vi "VISA Group WR.vi"(8 "error in (no error)":errorcluster, 10 "Array in":string[](array[string]), 11 "VISA Refnum in":refnum<visa-resource-name>) -> (0 "error out":errorcluster, 2 "Array out":string[](array[string]), 3 "VISA Refnum out":refnum<visa-resource-name>)   [LabVIEW 2014]
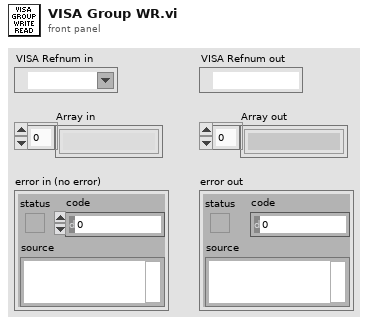
[diagram p1: front panel]
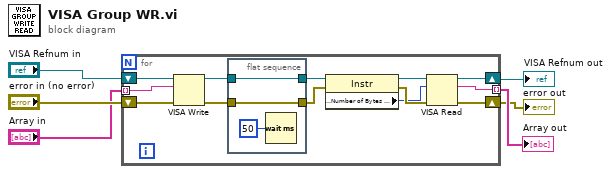
[diagram p0: block diagram]
diagram:
  n1 = for {
    tunnel: "Array in" -> [w19] mode=indexing
    tunnel: [w7] -> w6 mode=indexing
    shift-right: [w9] -> w4
    shift-left: "VISA Refnum in" -> [w18]
    shift-right: [w8] -> w5
    shift-left: "error in (no error)" -> [w16]
    n2 = VISA Write(VISA resource name=w18, write buffer=w19, error in (no error)=w16) -> (VISA resource name out=w17:refnum<visa-resource-name>, error out=w15:errorcluster)  [unwired: 1 out]
    n3 = flat-sequence {
      tunnel: w17 -> [w21]
      tunnel: w15 -> [w20]
      tunnel: [w21] -> w14
      tunnel: [w20] -> w13
      frame #0 {
        n4 = Wait (ms)(milliseconds to wait=u32 50) -> ()  [unwired: 1 out]
      }
    }
    n5 = property class="Instr"(reference=w14, error in=w13) -> (reference out=w12:refnum<visa-resource-name>, error out=w11:errorcluster, "Serial Settings:Number of Bytes at Serial Port"=w10:u32)
    n6 = VISA Read(VISA resource name=w12, byte count=w10, error in (no error)=w11) -> (VISA resource name out=w9:refnum<visa-resource-name>, read buffer=w7:string, error out=w8:errorcluster)  [unwired: 1 out]
  }
  "Array out" <- w6
  "error out" <- w5
  "VISA Refnum out" <- w4
